vi "OAT Color Map Indicator.vi"() -> ()   [LabVIEW 2017]
doc: "Uses Color Map to display results of spectral map on a customized intensity graph with a rainbow color scale."
uses:
  <vilib>/addons/Sound and Vibration/Order Analysis/Backward Compatibility/SubVIs/OAT Spectral Map.ctl
panel:
  out "Color Map":T1
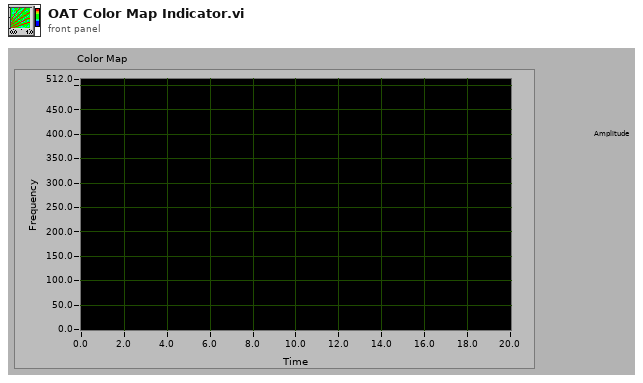
[diagram p1: front panel]
types:
  T1 = typedef "OAT Spectral Map.ctl" = dbl[][]
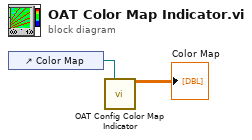
[diagram p0: block diagram]
diagram:
  n1 = control-ref of="Color Map"() -> (w1:refnum<vi>)
  n2 = call <vilib>:"OAT Config Color Map Indicator.vi"("color map ref"=w1) -> ("color map"=→"Color Map":T1)  [unwired: 13 in, 1 out]
